vi "Insert Image (ARGB with Greyscale Mask).vi"(6 "Greyscale Image Mask":T3, 7 "Offset (Default: 0,0)":T1, 8 "error in (no error)":errorcluster, 9 "ARGB Image Destination":T2, 10 "ARGB Image Child":T2, 11 "ARGB Image Parent":T2) -> (0 "error out":errorcluster, 3 "ARGB Image Destination (duplicate)":T2)   [LabVIEW 2020, in "g_ar_toolkit.image.lvlib"]
uses:
  g_ar_toolkit.image.lvlib
  ARGB Image.ctl
  Greyscale Image.ctl
  g_ar_toolkit.common/Image Point (Integer).ctl
  5e3288c8-ee88-4cfe-89cf-31ceca475f5a.vi
  g_ar_toolkit.common/Module Path.vi
  <vilib>/Utility/error.llb/Error Cluster From Error Code.vi
  g_ar_toolkit.common/g_ar_toolkit.common.lvlib
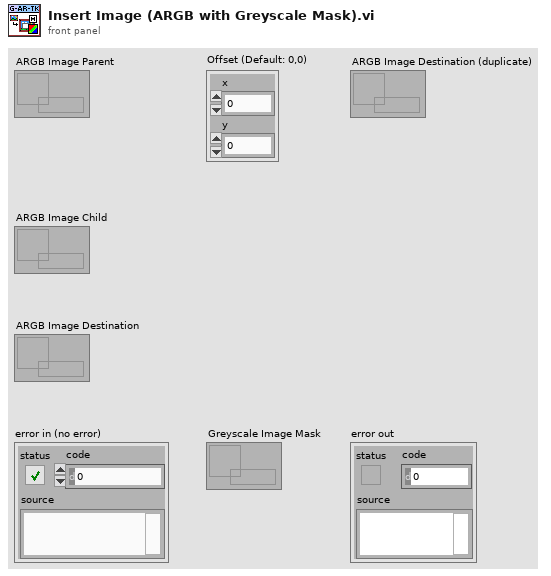
[diagram p1: front panel]
types:
  T1 = typedef "g_ar_toolkit.common.lvlib/Image Point (Integer).ctl" = cluster{"x":i32, "y":i32}
  T2 = typedef "g_ar_toolkit.image.lvlib/ARGB Image.ctl" = refnum<data-value>
  T3 = typedef "g_ar_toolkit.image.lvlib/Greyscale Image.ctl" = refnum<data-value>
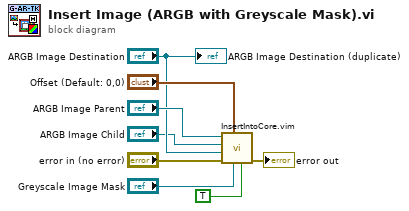
[diagram p0: block diagram]
diagram:
  n1 = call "InsertIntoCore.vim"("Has Mask"=TRUE, "Mask"="Greyscale Image Mask", "Offset"="Offset (Default: 0,0)", "error in (no error)"="error in (no error)", "Dst"="ARGB Image Destination", "Src_Child"="ARGB Image Child", "Src_Parent"="ARGB Image Parent") -> ("error out"=→"error out":errorcluster)  [unwired: 4 in]
  "ARGB Image Destination (duplicate)" <- "ARGB Image Destination"
